vi "Verify Type.vi"(8 "error in (no error)":errorcluster, 11 "CIF_CIPC_Chn_Double in":refnum<class "CIF_CIPC_Chn_Double.lvclass">) -> (0 "error out":errorcluster, 3 "CIF_CIPC_Chn_Double out":refnum<class "CIF_CIPC_Chn_Double.lvclass">)   [LabVIEW 2021, in "CIF_CIPC_Chn_Double.lvclass"]
uses:
  CIF_CIPC_Chn_Double.lvclass
  CIF_CIPC_Chn_Double.lvclass/CIF_CIPC_Chn_Double.ctl
  CIF_CIPC_Chan/CIF_CIPC_Chn.lvclass
  CIF_CIPC_Chan/Typedef/CIPC Channel Error.ctl
  <vilib>/Utility/Data Type/Type Definitions/Data Type.ctl
  <vilib>/Utility/Data Type/NI_Data Type.lvlib
  D:/dev/Packages/CIF_Channels_Core/src/CIPC_Channels/CIF_CIPC_Chan/CIF_CIPC_Chn.lvclass
  D:/dev/Packages/CIF_Channels_Core/src/CIFChannels/CIFChannels.lvclass
  D:/dev/Packages/CIF_Channels_Core/src/CIPC_Channels/double/CIF_CIPC_Chn_Double.lvclass
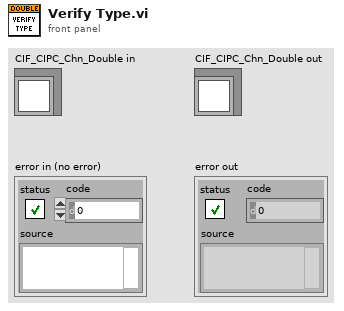
[diagram p1: front panel]
types:
  T1 = typedef "NI_Data Type.lvlib/Data Type.ctl" = enum8{"Invalid Type", "Void", "I8", "I16", "I32", "I64", "U8", "U16", "U32", "U64", "Single Float", "Double Float", "Extended Float", "Single Complex", "Double Complex", "Extended Complex", "Enum U8", "Enum U16", "Enum U32", "Enum U64", "Single Float With Unit", "Double Float With Unit", "Extended Float With Unit", "Single Complex with Unit", "Double Complex with Unit", "Extended Complex with Unit", "Boolean", "String", "Path", "Picture", "Tag", "Array", "Cluster", "Variant", "LV Variant", "Waveform", "Timestamp", "Digital Waveform", "Digital Data", "ExpressData", "Refnum", "External Data", "VI", "Poly VI", "LabVIEW Class Instance", "Fixed Point", "Set Collection", "Map Collection"}
  T2 = typedef "CIF_CIPC_Chn.lvclass/CIPC Channel Error.ctl" = enum16{"Type Mismatch"}
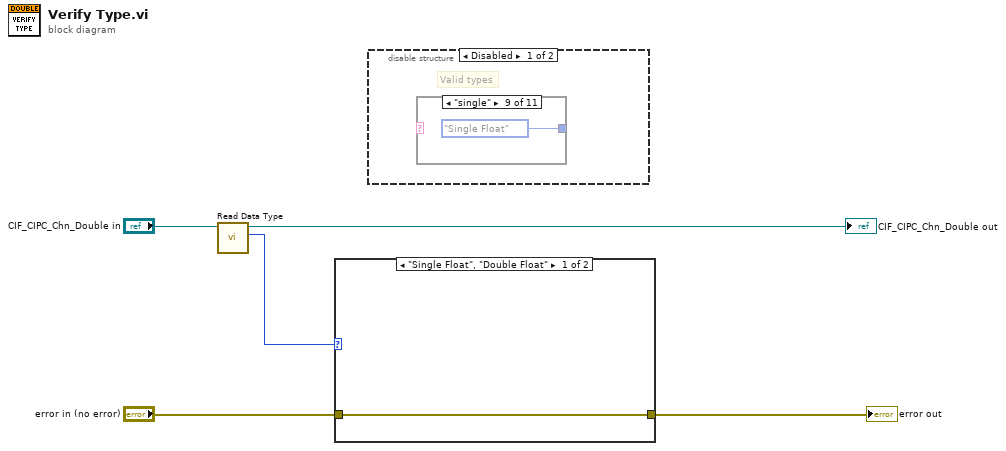
[diagram p0: block diagram]
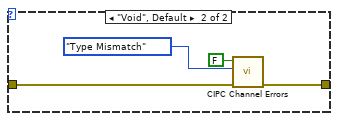
[diagram p2: hidden frame]
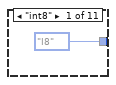
[diagram p3: hidden frame]
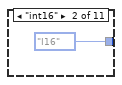
[diagram p4: hidden frame]
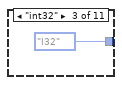
[diagram p5: hidden frame]
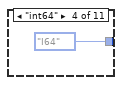
[diagram p6: hidden frame]
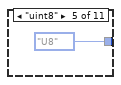
[diagram p7: hidden frame]
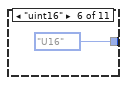
[diagram p8: hidden frame]
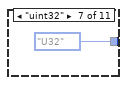
[diagram p9: hidden frame]
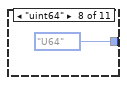
[diagram p10: hidden frame]
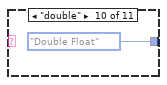
[diagram p11: hidden frame]
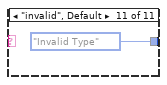
[diagram p12: hidden frame]
diagram:
  n1 = call "Read Data Type.vi"("CIF_CIPC_Chn in"="CIF_CIPC_Chn_Double in") -> ("Type Enum"=w1:T1, "CIF_CIPC_Chn out"=→"CIF_CIPC_Chn_Double out":refnum<class "CIF_CIPC_Chn_Double.lvclass">)  [unwired: 8 in, 1 out]
  n2 = case shown="\"Single Float\", \"Double Float\"" w1 {
    tunnel: "error in (no error)" -> [w6 w10]
    tunnel: [w6 w9] -> w4
    frame "Single Float", "Double Float" {
    }
    frame "Void", Default {
      n3 = call "CIPC Channel Errors.vi"("error in (no error)"=w10, "Error"=CIPC_Channel_Error."Type Mismatch", "Insert Error"=FALSE) -> ("error out"=w9:errorcluster)  [unwired: 8 in]
    }
  }
  "error out" <- w4
  n4 = disable-structure shown="Disabled" {
    frame Disabled {
      # "Valid types"
      n5 = case shown="\"single\"" {
        selector: _ -> [_ _ _ _ _ _ _ _ _ _ _]
        tunnel: [Data_Type."I8" ("Type") Data_Type."I16" ("Type") Data_Type."I32" ("Type") Data_Type."I64" ("Type") Data_Type."U8" ("Type") Data_Type."U16" ("Type") Data_Type."U32" ("Type") Data_Type."U64" ("Type") Data_Type."Single Float" ("Type") Data_Type."Double Float" ("Type") Data_Type."Invalid Type" ("Type")] -> _
        frame "int8" {
        }
        frame "int16" {
        }
        frame "int32" {
        }
        frame "int64" {
        }
        frame "uint8" {
        }
        frame "uint16" {
        }
        frame "uint32" {
        }
        frame "uint64" {
        }
        frame "single" {
        }
        frame "double" {
        }
        frame "invalid", Default {
        }
      }
    }
    frame Enabled {
    }
  }
